vi "RT_simul.vi"() -> ()   [LabVIEW 2011]
uses:
  <vilib>/platform/TimedLoop/XDataNode/XDataNode.xnode
  <vilib>/Platform/TimedLoop/XDataNode/nitl_modes.ctl
  <vilib>/Platform/TimedLoop/XDataNode/XDNodeRunTimeDep.lvlib
  <vilib>/Platform/TimedLoop/XDataNode/wakeup.ctl
  <vilib>/Platform/TimedLoop/XDataNode/timing_clust.ctl
  <vilib>/Utility/file.llb/Read Delimited Spreadsheet (DBL).vi
panel:
  out "End of simulation":bool
  out "t [s]":dbl
  in  "Simulation Time [s]":i32=85
  out "Iteration Duration":i64(graph)
  out "Data":dbl[][](array[numeric])
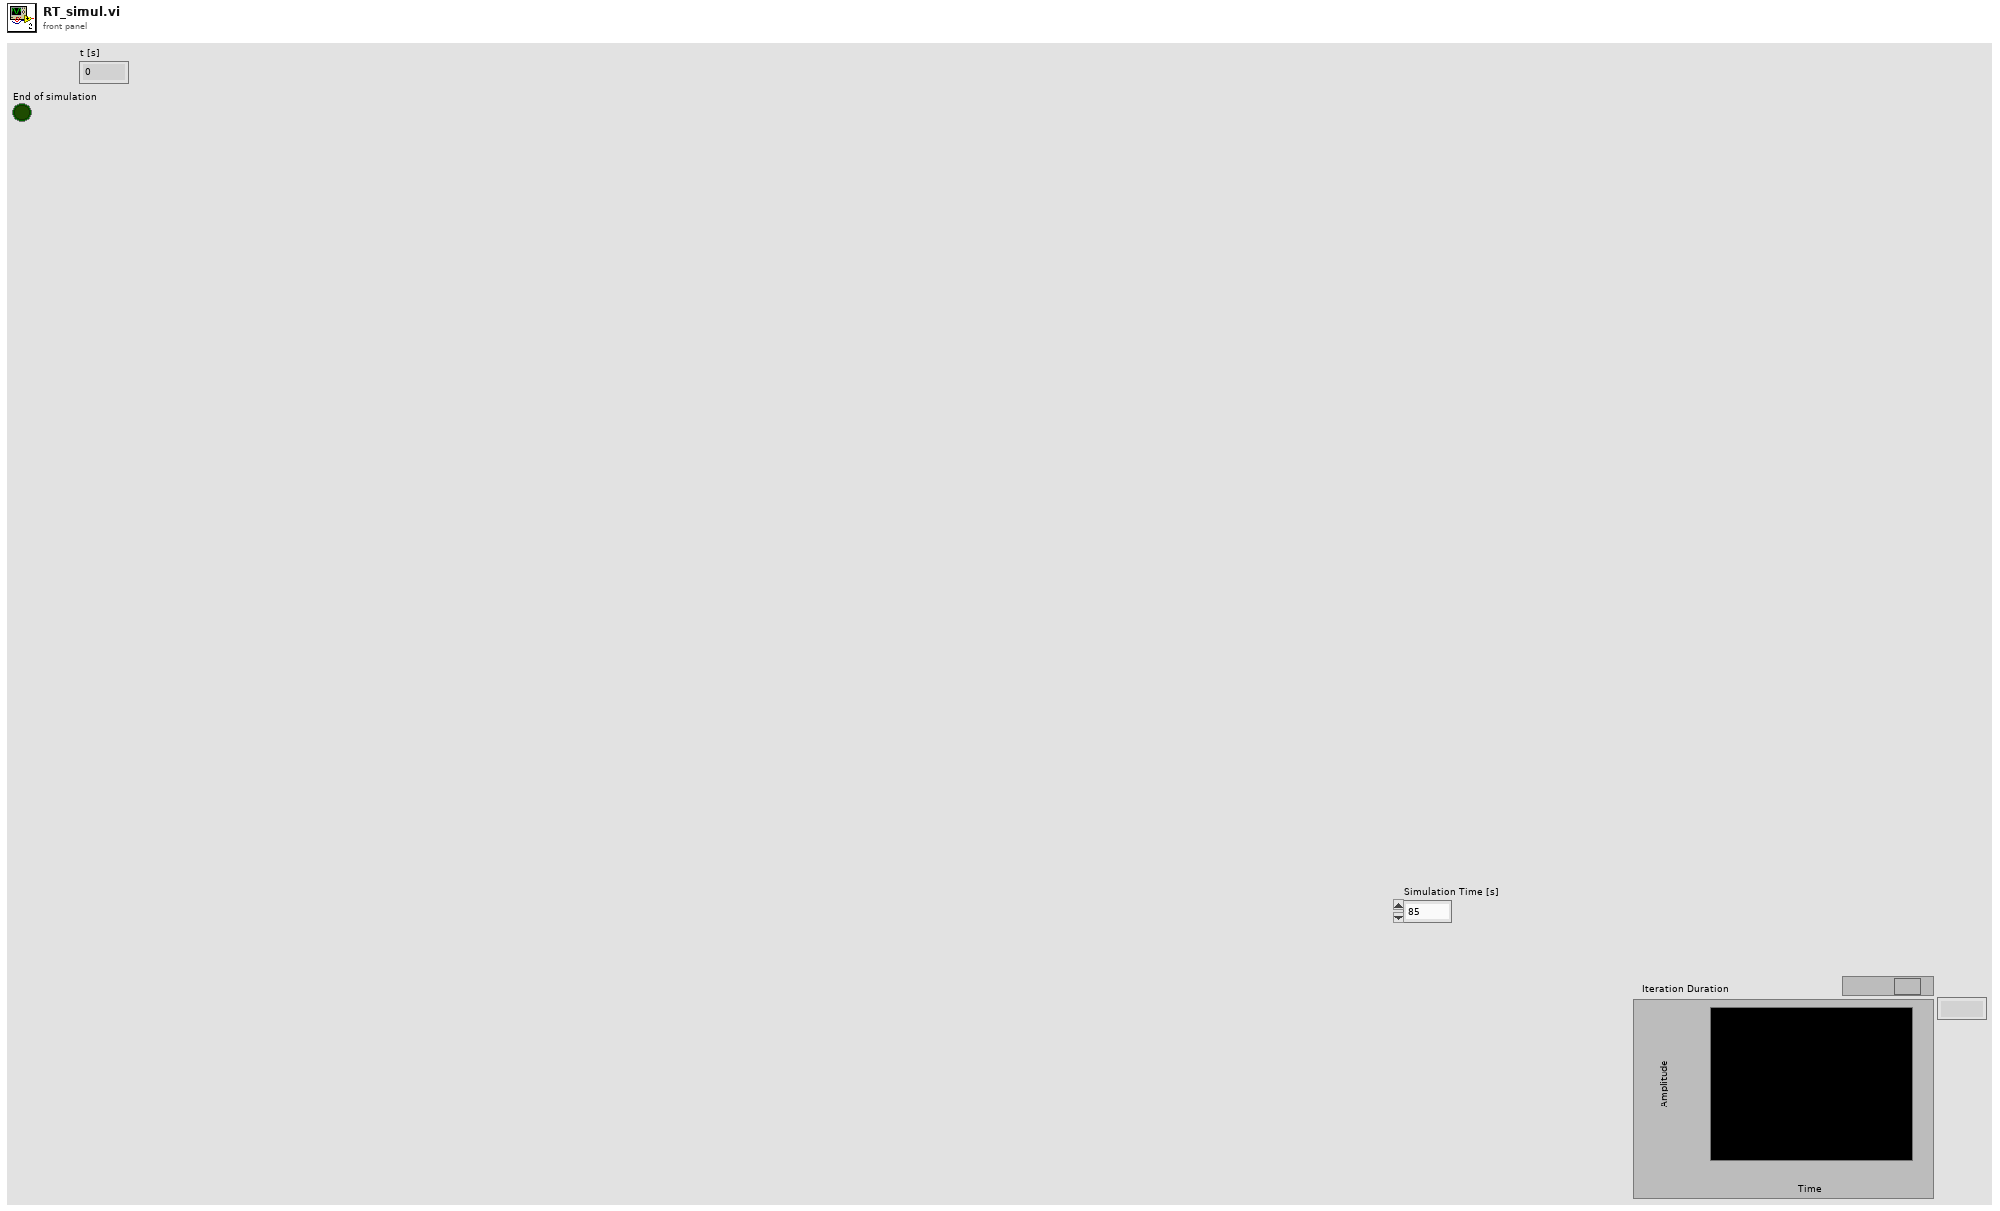
[diagram p1: front panel]
types:
  T1 = typedef "XDNodeRunTimeDep.lvlib/timing_clust.ctl" = cluster{"Expected End [f-1]":u64, "Actual End [f-1]":u64, "Finished Late? [f-1]":bool, "Expected End [i-1]":u64, "Actual End [i-1]":u64, "Finished Late? [i-1]":bool, "Expected Start [i]":u64, "Actual Start [i]":u64, "Expected Start [f]":u64, "Actual Start [f]":u64, "Source Name":string, "Structure Name":string, "Period":i64, "Deadline":i64, "Offset":i64, "Start":i64, "Priority":i32, "Timeout":i32, "Mode":T2, "Wakeup Reason":T3, "Error":errorcluster, "Source Type":string, "Secondary Source Type":string, "Global End Time":u64, "Global Start Time":u64, "Frame Duration":u64, "Iteration Duration":u64, "Assigned CPU":i32, "I/O Scan Engine Mode":u32}
  T2 = typedef "XDNodeRunTimeDep.lvlib/nitl_modes.ctl" = enum32{"No Change", "Process missed periods, maintain original phase", "Discard missed periods, maintain original phase", "Process missed periods, ignore original phase", "Discard missed periods, ignore original phase"}
  T3 = typedef "XDNodeRunTimeDep.lvlib/wakeup.ctl" = enum32{"Normal", "Aborted", "Asynchronous wakeup", "Timing source error", "Timed loop error", "Timeout"}
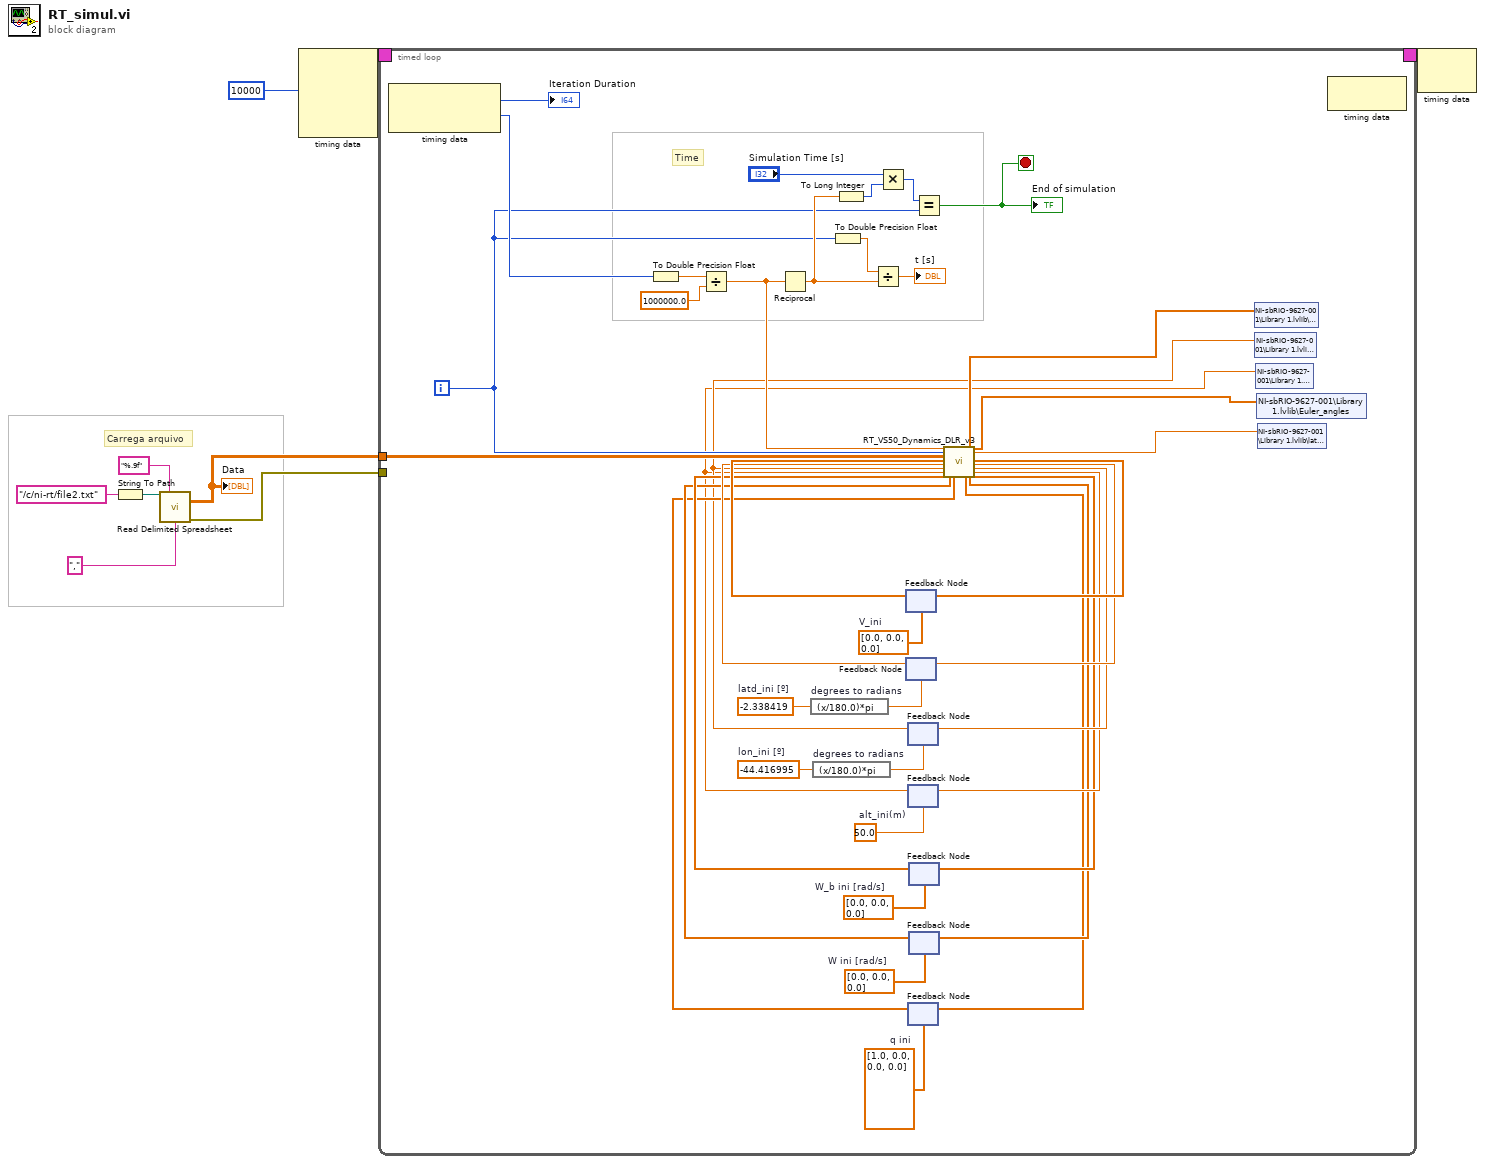
[diagram p0: block diagram]
diagram:
  # "Carrega arquivo"
  n1 = String To Path(string="/c/ni-rt/file2.txt") -> (path=w6:path)
  n2 = call-poly <vilib>:"Read Delimited Spreadsheet.vi"("file path (dialog if empty)"=w6, "format (%.3f)"="%.9f", "delimiter (\\t)"="," ("delimiter (\\t)")) -> ("all rows"=w1:dbl[][], "error out"=w4:errorcluster)  [unwired: 7 in, 4 out]
  "Data" <- w1
  n3 = node-c288(i64 10000 ("Period")) -> (w9:T1)  [unwired: 3 in]
  n4 = timed-loop {
    timing: w9 -> [_]
    timing-out: [_] -> w8
    tunnel: w1 -> [w27]
    tunnel: w4 -> [_]
    i -> [w28]
    stop <- w40 stop-if-true
    w30 = dbl[] [1.0, 0.0, 0.0, 0.0]  # q ini
    w31 = dbl[] [0.0, 0.0, 0.0]  # W_b ini [rad/s]
    w32 = dbl[] [0.0, 0.0, 0.0]  # W ini [rad/s]
    w37 = dbl[] [0.0, 0.0, 0.0]  # V_ini
    w38 = 50.0  # alt_ini(m)
    w36 = -44.416995  # lon_ini [º]
    w35 = -2.338419  # latd_ini [º]
    # "Time"
    n5 = node-c288() -> (→"Iteration Duration":i64, w41:i64)  [unwired: 1 in]
    n6 = To Double Precision Float(number=w41) -> (double precision float=w47:dbl)
    n7 = Divide(x=w47, y=1000000.0) -> (x/y=w29:dbl)
    n8 = Reciprocal(x=w29) -> (1/x=w44:dbl)
    n9 = expression code="(x/180.0)*pi" "degrees to radians"(w35) -> (w33:dbl)
    n10 = expression code="(x/180.0)*pi" "degrees to radians"(w36) -> (w34:dbl)
    n11 = To Double Precision Float(number=w28) -> (double precision float=w43:dbl)
    n12 = To Long Integer(number=w44) -> (32bit integer=w45:i32)
    n13 = Divide(x=w43, y=w44) -> (x/y=→"t [s]":dbl)
    n14 = Multiply(x="Simulation Time [s]", y=w45) -> (x*y=w48:i32)
    n15 = feedback #1(w37) -> (w26:dbl[])
    n16 = feedback #2(w33) -> (w25:dbl)
    n17 = feedback #3(w34) -> (w11:dbl)
    n18 = feedback #4(w38) -> (w10:dbl)
    n19 = feedback #5(w30) -> (w22:dbl[])
    n20 = feedback #6(w31) -> (w24:dbl[])
    n21 = feedback #7(w32) -> (w23:dbl[])
    n22 = Equal?(x=w48, y=w28) -> (x = y?=w40:bool)
    "End of simulation" <- w40
    n23 = call "RT_VS50_Dynamics_DLR_v3.vi"("dt [s]"=w29, "i"=w28, "Data"=w27, "V(i) [m/s]"=w26, "latd(i) [rad]"=w25, "lon(i) [rad]"=w11, "alt(i)[m]"=w10, "W_b(i) [rad/s]"=w24, "W(i) [rad/s]"=w23, "q(i)"=w22) -> ("q(i+1) 2"=w13:dbl[], "P(i) [m]"=w12:dbl[], "W(i+1) [rad/s]"=w14:dbl[], "Euler Angles (º)"=w21:dbl[], "L_C"=w20:dbl, "V(i+1) [m/s]"=w19:dbl[], "latd(i+1) [rad]"=w18:dbl, "lon(i+1)[rad]"=w17:dbl, "alt(i+1) [m]"=w16:dbl, "W_b(i+1) [rad/s]"=w15:dbl[])  [unwired: 8 in]
    n24 = feedback-in #1(w19) -> ()
    n25 = feedback-in #2(w18) -> ()
    n26 = feedback-in #3(w17) -> ()
    n27 = feedback-in #4(w16) -> ()
    n28 = feedback-in #5(w13) -> ()
    n29 = feedback-in #6(w15) -> ()
    n30 = feedback-in #7(w14) -> ()
    n31 = shared-variable "NI-sbRIO-9627-001\\Library 1.lvlib\\Pos"(w12) -> ()  [unwired: 1 in, 1 out]
    n32 = shared-variable "NI-sbRIO-9627-001\\Library 1.lvlib\\lon"(w11) -> ()  [unwired: 1 in, 1 out]
    n33 = shared-variable "NI-sbRIO-9627-001\\Library 1.lvlib\\alt"(w10) -> ()  [unwired: 1 in, 1 out]
    n34 = shared-variable "NI-sbRIO-9627-001\\Library 1.lvlib\\Euler_angles"(w21) -> ()  [unwired: 1 in, 1 out]
    n35 = shared-variable "NI-sbRIO-9627-001\\Library 1.lvlib\\lat_c"(w20) -> ()  [unwired: 1 in, 1 out]
    n36 = node-c288() -> ()  [unwired: 1 in, 1 out]
  }
  n37 = node-c288(w8) -> ()  [unwired: 1 out]
